vi "ClassObtainRefs.vi"(8 "error in":errorcluster, 10 "Class Name":string="Class 1") -> (0 "error out":errorcluster, 3 "Ref cluster":T1)   [LabVIEW 2025, in "UI_Library.lvlib" / "UI_Library.lvclass"]
doc: "Obtain the references of all the controls of the Class private data"
uses:
  UI_Library.lvclass
  Controls/UI_RefCluster.ctl
  <vilib>/Utility/Data Type/Type Definitions/Data Type.ctl
  <vilib>/Utility/Data Type/NI_Data Type.lvlib
  UI_Library.lvlib
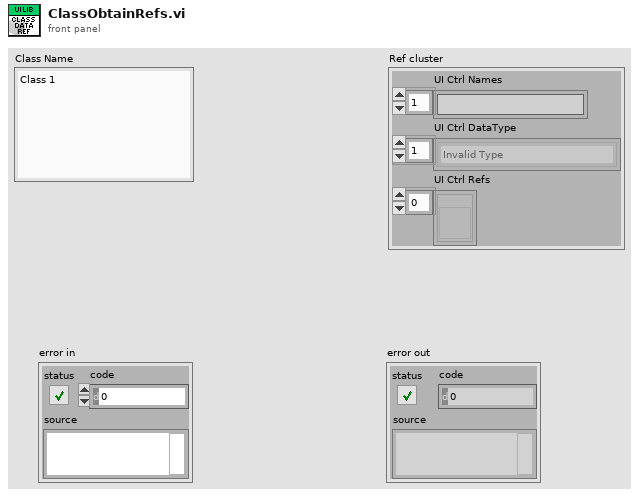
[diagram p1: front panel]
types:
  T1 = typedef "UI_Library.lvlib/UI_RefCluster.ctl" = cluster{"UI Ctrl Names":string[], "UI Ctrl DataType":T2[], "UI Ctrl Refs":refnum<vi>[]}
  T2 = typedef "NI_Data Type.lvlib/Data Type.ctl" = enum8{"Invalid Type", "Void", "I8", "I16", "I32", "I64", "U8", "U16", "U32", "U64", "Single Float", "Double Float", "Extended Float", "Single Complex", "Double Complex", "Extended Complex", "Enum U8", "Enum U16", "Enum U32", "Enum U64", "Single Float With Unit", "Double Float With Unit", "Extended Float With Unit", "Single Complex with Unit", "Double Complex with Unit", "Extended Complex with Unit", "Boolean", "String", "Path", "Picture", "Tag", "Array", "Cluster", "Variant", "LV Variant", "Waveform", "Timestamp", "Digital Waveform", "Digital Data", "ExpressData", "Refnum", "External Data", "VI", "Poly VI", "LabVIEW Class Instance", "Fixed Point", "Set Collection", "Map Collection"}
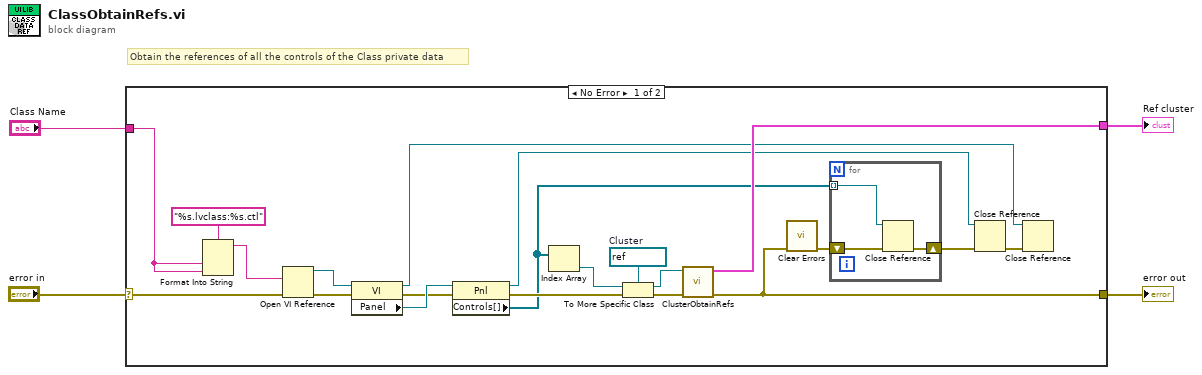
[diagram p0: block diagram]
diagram:
  # "Obtain the references of all the controls of the Class private data"
  n1 = case shown="No Error" "error in" {
    selector: "error in" -> [w16 w29]
    tunnel: "Class Name" -> [w22 _]
    tunnel: [w17 _] -> w3
    tunnel: [w5 w29] -> w1
    frame No Error {
      w18 = refnum<vi> refnum  # Cluster
      n2 = Format Into String(format string="%s.lvclass:%s.ctl", w22, w22) -> (resulting string=w23:string)  [unwired: 2 in, 1 out]
      n3 = Open VI Reference(vi path=w23, error in (no error)=w16) -> (vi reference=w21:refnum<vi>, error out=w15:errorcluster)  [unwired: 4 in]
      n4 = property on="Property Node" class="VI"(reference=w21, error in=w15) -> (reference out=w7:refnum<vi>, error out=w13:errorcluster, "Panel"=w25:refnum<vi>)
      n5 = property on="Property Node" class="Pnl"(reference=w25, error in=w13) -> (reference out=w8:refnum<vi>, error out=w12:errorcluster, "Controls[]"=w9:refnum<vi>[])
      n6 = Index Array(array=w9) -> (element=w20:refnum<vi>)  [unwired: 1 in]
      n7 = To More Specific Class(target class=w18, reference=w20, error in=w12) -> (specific class reference=w19:refnum<vi>, error out=w14:errorcluster)
      n8 = call "ClusterObtainRefs.vi"("error in (no error)"=w14, "Clust Refnum"=w19) -> ("error out"=w5:errorcluster, "Ref cluster"=w17:T1)  [unwired: 8 in]
      n9 = call <vilib>:"Clear Errors.vi"("error in (no error)"=w5) -> ("error out"=w6:errorcluster)  [unwired: 5 in, 1 out]
      n10 = for {
        tunnel: w9 -> [w26] mode=indexing
        shift-right: [w27] -> w11
        shift-left: w6 -> [w28]
        n11 = Close Reference(reference=w26, error in (no error)=w28) -> (error out=w27:errorcluster)
      }
      n12 = Close Reference(reference=w8, error in (no error)=w11) -> (error out=w10:errorcluster)
      n13 = Close Reference(reference=w7, error in (no error)=w10) -> ()  [unwired: 1 out]
    }
    frame Error {
    }
  }
  "Ref cluster" <- w3
  "error out" <- w1
